vi "FPGA Read FIFO By Name.vi"   [LabVIEW 2010, in "FPGA Interface Base.lvclass"]
doc: "Reads data from a FIFO"
uses:
  <userlib>/_FPGA Interface Advanced Tools/FPGA Interface Base/FPGA Interface Base.lvclass
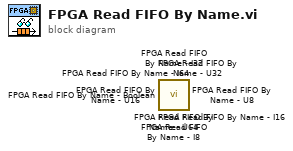
[diagram p0: block diagram]
diagram:
  n1 = call <userlib>:"FPGA Read FIFO By Name - U64.vi"() -> ()  [unwired: 8 in, 4 out]
  n2 = call <userlib>:"FPGA Read FIFO By Name - U32.vi"() -> ()  [unwired: 8 in, 4 out]
  n3 = call <userlib>:"FPGA Read FIFO By Name - U16.vi"() -> ()  [unwired: 8 in, 4 out]
  n4 = call <userlib>:"FPGA Read FIFO By Name - U8.vi"() -> ()  [unwired: 8 in, 4 out]
  n5 = call <userlib>:"FPGA Read FIFO By Name - I64.vi"() -> ()  [unwired: 8 in, 4 out]
  n6 = call <userlib>:"FPGA Read FIFO By Name - I32.vi"() -> ()  [unwired: 8 in, 4 out]
  n7 = call <userlib>:"FPGA Read FIFO By Name - I16.vi"() -> ()  [unwired: 8 in, 4 out]
  n8 = call <userlib>:"FPGA Read FIFO By Name - I8.vi"() -> ()  [unwired: 8 in, 4 out]
  n9 = call <userlib>:"FPGA Read FIFO By Name - Boolean.vi"() -> ()  [unwired: 8 in, 4 out]
